vi "Write Parent Hwnd.vi"(8 "error in (no error)":errorcluster, 10 "Parent Hwnd":i32, 11 "LV MDI in":refnum<class "LV MDI.lvclass">) -> (0 "error out":errorcluster, 3 "LV MDI out":refnum<class "LV MDI.lvclass">)   [LabVIEW 2019, in "LV MDI.lvclass"]
uses:
  LV MDI.lvclass
  LV MDI.lvclass/LV MDI.ctl
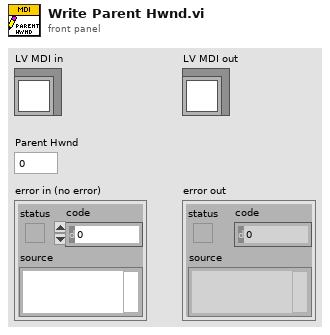
[diagram p1: front panel]
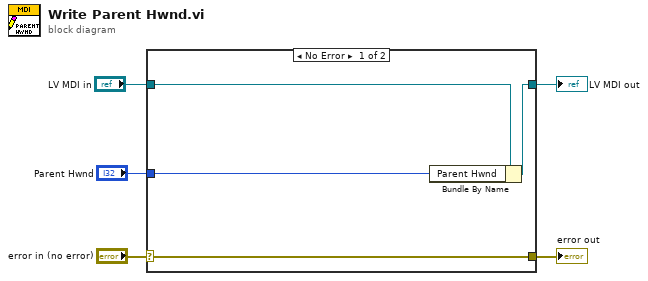
[diagram p0: block diagram]
diagram:
  n1 = case shown="No Error" "error in (no error)" {
    selector: "error in (no error)" -> [w9 w10]
    tunnel: [w9 w10] -> w4
    tunnel: [w7 w11] -> w2
    tunnel: "LV MDI in" -> [w8 w11]
    tunnel: "Parent Hwnd" -> [w6 _]
    frame No Error {
      n2 = Bundle By Name(cluster=w8, "Parent Hwnd"=w6) -> (w7:refnum<class "LV MDI.lvclass">)
    }
    frame Error {
    }
  }
  "error out" <- w4
  "LV MDI out" <- w2
